vi "Set_MultiVar_Value.vi"(8 "error in (no error)":errorcluster, 9 "varValue":dbl format="%#_13g", 10 "varName":string, 11 "mupExpr in":refnum<data-value>) -> (0 "error out":errorcluster, 3 "mupExpr out":refnum<data-value>)   [LabVIEW 2015, in "mupExpr.lvclass"]
doc: "Set the value of the specified variable variable.\n\nIf the variable is not found, a warning is generated."
uses:
  mupExpr.lvclass
  mupExpr.lvclass/mupExpr.ctl
  mupLib/mupSetVarValue.vi
  <vilib>/Utility/error.llb/Error Cluster From Error Code.vi
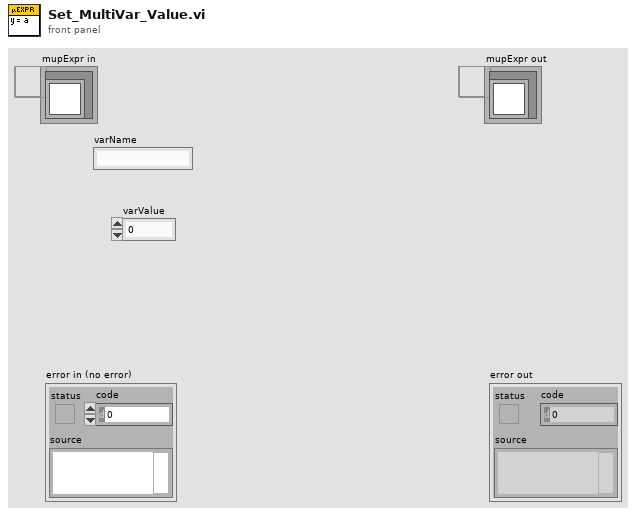
[diagram p1: front panel]
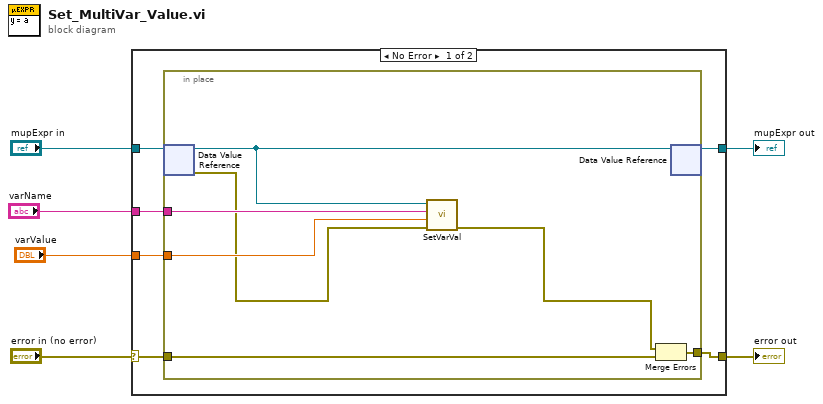
[diagram p0: block diagram]
diagram:
  n1 = case shown="No Error" "error in (no error)" {
    selector: "error in (no error)" -> [w7 w20]
    tunnel: "varValue" -> [w12 _]
    tunnel: "varName" -> [w11 _]
    tunnel: "mupExpr in" -> [w10 w21]
    tunnel: [w9 w20] -> w3
    tunnel: [w8 w21] -> w2
    frame No Error {
      n2 = in-place {
        in-place-border: w7 -> [w15]
        in-place-border: w12 -> [w19]
        in-place-border: w11 -> [w18]
        in-place-border: [w14] -> w9
        n3 = in-place-dvr #1(w10) -> (w13:refnum<class "mupExpr.lvclass">, w17:errorcluster)
        n4 = call "SetVarVal.vi"("error in (no error)"=w17, "varValue"=w19, "varName"=w18, "muExpr in"=w13) -> ("error out"=w16:errorcluster)  [unwired: 6 in, 1 out]
        n5 = Merge Errors(w16, w15) -> (w14:errorcluster)
        n6 = in-place-dvr #1(w13) -> (w8:refnum<data-value>)  [unwired: 1 out]
      }
    }
    frame Error {
    }
  }
  "error out" <- w3
  "mupExpr out" <- w2
